vi "4145_About.vi"() -> ()   [LabVIEW 2014]
panel:
  in  "Boolean":bool
  # "HP 4145 data gathering utility\nVersion 1.0"
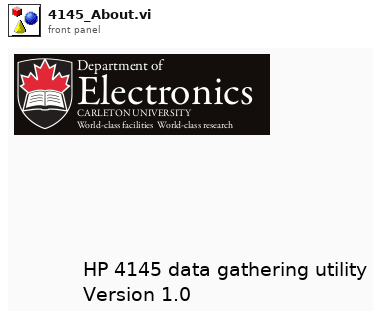
[diagram p1: front panel]
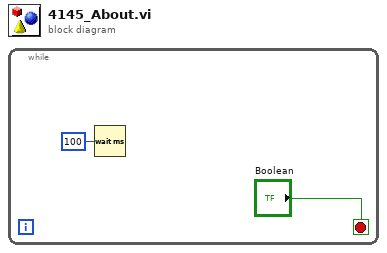
[diagram p0: block diagram]
diagram:
  n1 = while {
    stop <- "Boolean" stop-if-true
    n2 = Wait (ms)(milliseconds to wait=u32 100) -> ()  [unwired: 1 out]
  }
